vi "SL TAGS Return Tags of Type.vi"(8 "error in (no error)":errorcluster, 9 "Tag Type":T1, 11 "EEISysLink in":refnum<class "EEISysLink.lvclass">) -> (0 "error out":errorcluster, 2 "Tags of Type":T2[](array[typedef]), 3 "EEISysLink out":refnum<class "EEISysLink.lvclass">)   [LabVIEW 2017, in "EEISysLink.lvclass"]
doc: "Will input an array of class tags and return all of them that match a type. \n\nJames Tillett P.E.\nEndeavor Engineering Inc.\nwww.endeavoreng.com"
uses:
  EEISysLink.lvclass
  Controls/SL Tag.ctl
  <vilib>/Skyline/Tag/Wrapper/Wrapper_class/NI Skyline Tag.lvclass
  Controls/SL Tag Properties.ctl
  Controls/SL Tag Data Type.ctl
  Controls/SL Tag Interpolation Method.ctl
  Controls/SL Tag Unit of Measure.ctl
  Controls/SL Tag Type.ctl
  <vilib>/Skyline/Tag/Shared/typedefs/Tag Cluster.ctl
  <vilib>/Skyline/Tag/Shared/typedefs/DataType.ctl
  EEISysLink.lvclass/EEISysLink.ctl
  <vilib>/Skyline/Tag/Wrapper/Wrapper_class/Read Tag (I32).vi
  <vilib>/Skyline/Tag/Wrapper/Wrapper_class/Read Tag (DBL).vi
  <vilib>/Skyline/Tag/Shared/NI Skyline Tag.lvlib
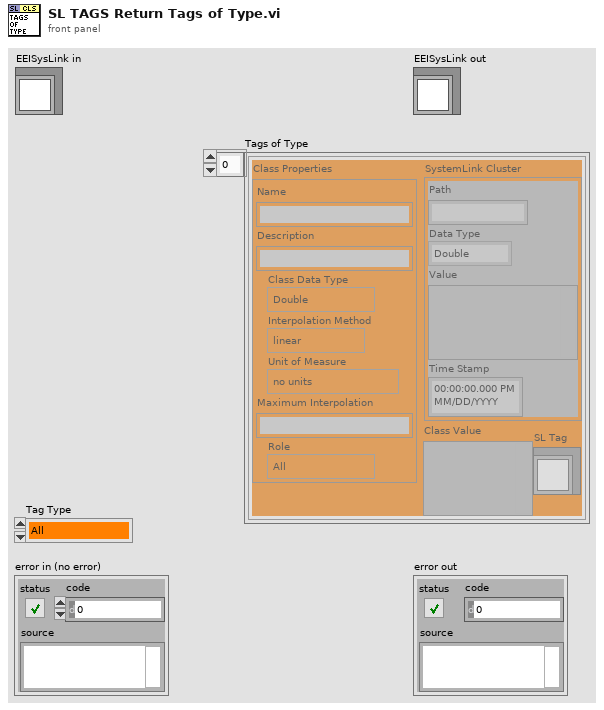
[diagram p1: front panel]
types:
  T1 = typedef "EEISysLink.lvclass/SL Tag Type.ctl" = enum16{"All", "Supervisor", "Worker"}
  T2 = typedef "EEISysLink.lvclass/SL Tag.ctl" = cluster{"Class Properties":T3, "SL Tag":refnum<class "NI Skyline Tag.lvclass">, "SystemLink Cluster":T7, "Class Value":variant}
  T3 = typedef "EEISysLink.lvclass/SL Tag Properties.ctl" = cluster{"Class Data Type":T4, "Name":string, "Description":string, "Interpolation Method":T5, "Unit of Measure":T6, "Maximum Interpolation":string, "Role":T1}
  T4 = typedef "EEISysLink.lvclass/SL Tag Data Type.ctl" = enum16{"Double", "Integer", "String", "Boolean", "Waveform"}
  T5 = typedef "EEISysLink.lvclass/SL Tag Interpolation Method.ctl" = enum16{"linear", "pilinear", "step"}
  T6 = typedef "EEISysLink.lvclass/SL Tag Unit of Measure.ctl" = enum16{"no units", "Second", "Hour", "Minute", "Day", "Year", "Month", "Week", "Foot", "Yard", "Meter", "Centimeter", "Inch", "Mile", "Nautical Mile", "Miles per Hour", "Meters per second", "Square meter", "Cubic meter", "Cubic centimeter", "Cubic inch", "Liter", "Gallon", "Gallons dry US", "Gallon UK", "Percent", "Revolutions per minute", "Revolution", "Degree angle", "Astronomical Unit", "Atom", "Atomic mass", "Bar", "Byte", "C (speed of light)", "Curie", "Decibel", "Electron Volt", "Ounce", "Knot", "G", "Grade", "Are", "Hectare", "Faraday", "Franklin", "Gilbert", "Erg", "Lambert", "Maxwell", "Gauss", "Electron mass", "Kilogram force", "Pound force", "Rad", "Centiradian", "Sphere", "Mach", "Fluid Ounces", "Fluid Ounces UK", "Fahrenheit", "Celsius", "Kelvin", "Rankine", "Gram", "Kilogram", "Pound", "Short/US Ton", "Long/UK ton", "Metric ton", "Mole", "Pounds per square inch", "Inches water column", "Torr", "Millitorr", "Millimeter mercury", "Inches mercury", "Bar (2)", "Atmosphere", "Pascal", "Watt", "kiloWatt", "Horsepower", "Kilowatt Hour", "British thermal units", "Millions of BTU", "Ampere", "Candela", "Radian", "Steradian", "Bit", "Hertz", "Newton", "Joule", "Coulomb", "Volt", "Farad", "Ohm", "Siemens", "Weber", "Tesla", "Henry", "Lumen", "Lux", "Becqueral", "Gray", "Sievert", "Katal", "Angstrom", "Light Year", "Parsec", "Point", "Pixel", "Dyne", "Kilogram force (2)", "Pound force (2)", "Rem", "Rutherford", "Roentgen"}
  T7 = typedef "NI Skyline Tag.lvlib/Tag Cluster.ctl" = cluster{"Path":string, "Data Type":T8, "Value":variant, "Time Stamp":timestamp}
  T8 = typedef "NI Skyline Tag.lvlib/DataType.ctl" = enum32{"Double", "Integer", "String"}
  T9 = typedef "NI Skyline Tag.lvlib/Aggregates Int.ctl" = cluster{"Count":i32, "Max":i32, "Min":i32, "Mean":dbl}
  T10 = typedef "NI Skyline Tag.lvlib/Aggregates Double.ctl" = cluster{"Count":i32, "Max":dbl, "Min":dbl, "Mean":dbl}
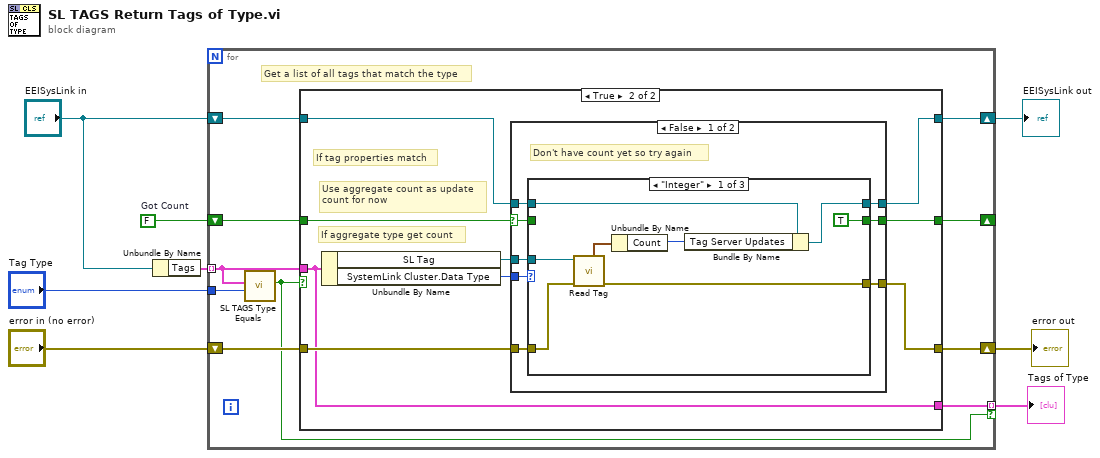
[diagram p0: block diagram]
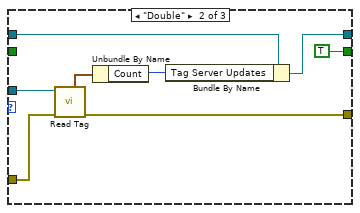
[diagram p3: hidden frame]
diagram:
  w4 = FALSE  # Got Count
  n1 = Unbundle By Name("EEISysLink in") -> ("Tags"=w1:T2[])
  n2 = for {
    tunnel: w1 -> [w18] mode=indexing
    tunnel: "Tag Type" -> [w17]
    shift-right: [w11] -> _
    shift-left: w4 -> [w15]
    shift-right: [w13] -> w6
    shift-left: "EEISysLink in" -> [w14]
    shift-right: [w12] -> w5
    shift-left: "error in (no error)" -> [w16]
    tunnel: [w10] -> w8 mode=indexing if=w9
    # "Get a list of all tags that match the type"
    n3 = call "SL TAGS Type Equals.vi"("Tag Type"=w17, "Tag"=w18) -> ("Match?"=w9:bool)  [unwired: 9 in]
    n4 = case shown="True" w9 {
      tunnel: w18 -> [_ w22]
      tunnel: w16 -> [w19 w29]
      tunnel: w15 -> [w21 w23]
      tunnel: [w21 w28] -> w11
      tunnel: w14 -> [w20 w27]
      tunnel: [w20 w26] -> w13
      tunnel: [w19 w25] -> w12
      tunnel: [_ w22] -> w10
      frame False {
        # "Type doesn't match so don't include"
      }
      frame True {
        # "If aggregate type get count"
        # "Use aggregate count as update\ncount for now"
        # "If tag properties match"
        n5 = Unbundle By Name(w22) -> ("SL Tag"=w24:refnum<class "NI Skyline Tag.lvclass">, "SystemLink Cluster.Data Type"=w30:T8)
        n6 = case shown="False" w23 {
          selector: w23 -> [w31 w59]
          tunnel: w30 -> [w38 _]
          tunnel: w29 -> [w37 w58]
          tunnel: [w36 w59] -> w28
          tunnel: w27 -> [w35 w60]
          tunnel: [w34 w60] -> w26
          tunnel: [w33 w58] -> w25
          tunnel: w24 -> [w32 _]
          frame False {
            # "Don't have count yet so try again"
            n7 = case shown="\"Integer\"" w38 {
              tunnel: w32 -> [w46 w54 _]
              tunnel: w37 -> [w45 w53 w57]
              tunnel: [w44 w52 w57] -> w33
              tunnel: w31 -> [_ _ w56]
              tunnel: [TRUE ("Got Count") TRUE ("Got Count") w56] -> w36
              tunnel: w35 -> [w41 w49 w55]
              tunnel: [w39 w47 w55] -> w34
              frame "Integer" {
                n8 = call-poly <vilib>:"Read Tag.vi"("error in (no error)"=w45, "tag in"=w46) -> ("error out"=w44:errorcluster, "Aggregate Values"=w43:T9)  [unwired: 5 in, 3 out]
                n9 = Unbundle By Name(w43) -> ("Count"=w40:i32)
                n10 = Bundle By Name(cluster=w41, "Tag Server Updates"=w40) -> (w39:refnum<class "EEISysLink.lvclass">)
              }
              frame "Double" {
                n11 = call-poly <vilib>:"Read Tag.vi"("error in (no error)"=w53, "tag in"=w54) -> ("error out"=w52:errorcluster, "Aggregate Values"=w51:T10)  [unwired: 5 in, 3 out]
                n12 = Unbundle By Name(w51) -> ("Count"=w48:i32)
                n13 = Bundle By Name(cluster=w49, "Tag Server Updates"=w48) -> (w47:refnum<class "EEISysLink.lvclass">)
              }
              frame "String" {
                # "String doesn't return aggregates so don't use for count"
              }
            }
          }
          frame True {
            # "Already got the count so don't need more"
          }
        }
      }
    }
  }
  "Tags of Type" <- w8
  "EEISysLink out" <- w6
  "error out" <- w5
